vi "CCD shot image.vi"(6 "CCD GPIB Address":u16=1, 9 "Shutter Enabled":bool=TRUE, 10 "Exposuretime (s)":dbl=0.5 format="%.2f") -> (1 "#PixelOverflow":u32, 2 "PixelOverflow":bool, 3 "Intensity graph":i32[][](graph), 5 "Setup String":string="ldu,0,256,16;sdu,0,1024,1024;cl0;omrm;sron")   [LabVIEW 2019]
doc: "This VI demonstrates how to interactively create a color table for an intensity graph. This VI uses color table generator as a subVI to allow the user to create a new color table.\n\n_KEYWORDS_: intensity graph, color table, color array"
panel:
  in  "Recalculate data":bool
  in  "Set back to array":bool
  in  "Generate color table":bool
  in  "Stop button":bool=TRUE
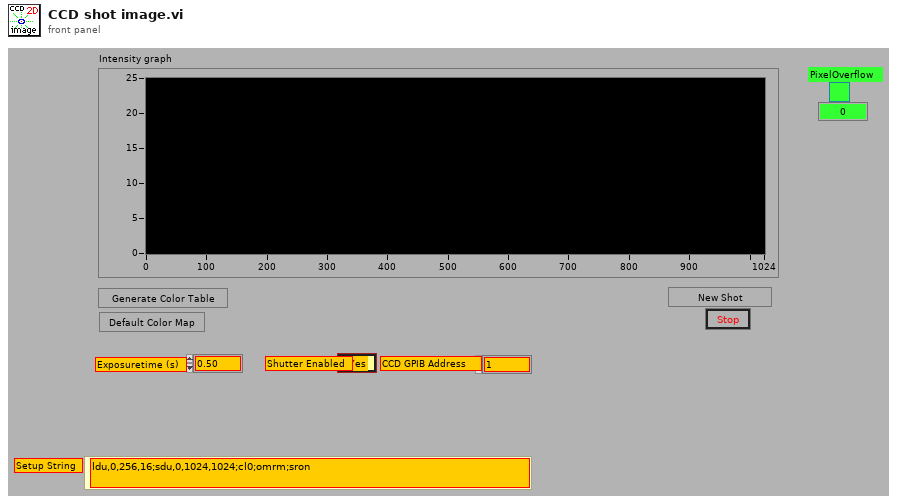
[diagram p1: front panel]
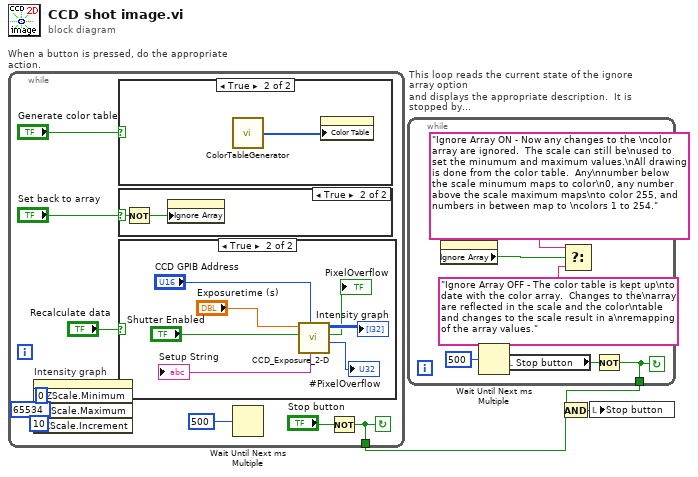
[diagram p0: block diagram]
diagram:
  n1 = while "When a button is pressed, do the appropriate action." {
    tunnel: [w5] -> w3
    stop <- w5 continue-if-true
    n2 = property on="Intensity graph" class="IntGraph (strict)"("ZScale.Minimum"=u32 0 ("Z Minimum"), "ZScale.Maximum"=u32 65534 ("Z Maximum"), "ZScale.Increment"=u32 10 ("Z Increment")) -> ()  [unwired: 2 in, 2 out]
    n3 = case shown="True" "Generate color table" {
      frame False {
      }
      frame True {
        n4 = call "ColorTableGenerator.vi"() -> (w22:u32[])
        n5 = property on="Intensity graph" class="IntGraph (strict)"("Color Table"=w22) -> ()  [unwired: 2 in, 2 out]
      }
    }
    n6 = case shown="True" "Set back to array" {
      selector: "Set back to array" -> [_ w21]
      frame False {
      }
      frame True {
        n7 = Not(x=w21) -> (.not. x?=w20:bool)
        n8 = property class="IntGraph (strict)"("Ignore Array"=w20) -> ()  [unwired: 2 in, 2 out]
      }
    }
    n9 = case shown="True" "Recalculate data" {
      frame False {
      }
      frame True {
        n10 = call "CCD_Exposure_2-D.vi"("CCD GPIB Address"="CCD GPIB Address", "Shutter Enabled"="Shutter Enabled", "Exposuretime (s)"="Exposuretime (s)") -> ("#PixelOverflow"=→"#PixelOverflow":u32, "PixelOverflow"=→"PixelOverflow":bool, "The Data"=→"Intensity graph":i32[][], "Setup String"=→"Setup String":string)  [unwired: 2 in, 3 out]
      }
    }
    n11 = Wait Until Next ms Multiple(millisecond multiple=u32 500) -> ()  [unwired: 1 out]
    n12 = Not(x="Stop button") -> (.not. x?=w5:bool)
  }
  n13 = while "This loop reads the current state of the ignore array option\nand displays the appropriate description.  It is stopped by\nreading a local on the stop button." {
    tunnel: [w24] -> w2
    stop <- w24 continue-if-true
    n14 = property on="Intensity graph" class="IntGraph (strict)"() -> ("Ignore Array"=w28:bool)  [unwired: 2 in, 2 out]
    n15 = Wait Until Next ms Multiple(millisecond multiple=u32 500) -> ()  [unwired: 1 out]
    n16 = local read "Stop button"() -> (w23:bool)
    n17 = Select(t="Ignore Array ON - Now any changes to the \ncolor array are ignored.  The scale can still be\nused to set the minumum and maximum values.\nAll drawing is done from the color table.  Any\nnumber below the scale minumum maps to color\n0, any number above the scale maximum maps\nto color 255, and numbers in between map to \ncolors 1 to 254.", s=w28, f="Ignore Array OFF - The color table is kept up\nto date with the color array.  Changes to the\narray are reflected in the scale and the color\ntable and changes to the scale result in a\nremapping of the array values.") -> ()  [unwired: 1 out]
    n18 = Not(x=w23) -> (.not. x?=w24:bool)
  }
  n19 = And(x=w2, y=w3) -> (x .and. y?=w1:bool)
  n20 = local write "Stop button"(w1) -> ()
